vi "Delay.vi"(8 "error in (no error)":errorcluster, 10 "Delay Time (50 ms)":u32=50, 11 "VISA resource name":refnum<visa-resource-name>="TCPIP0::192.168.0.200::50505::SOCKET") -> (0 "error out":errorcluster, 3 "VISA resource name out":refnum<visa-resource-name>="TCPIP0::192.168.0.200::50505::SOCKET")   [LabVIEW 2022 SP3, in "MagnaDC.lvlib"]
uses:
  MagnaDC.lvlib
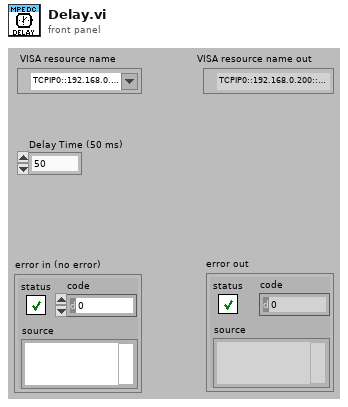
[diagram p1: front panel]
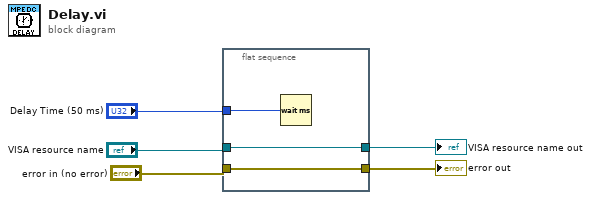
[diagram p0: block diagram]
diagram:
  n1 = flat-sequence {
    tunnel: "Delay Time (50 ms)" -> [w8]
    tunnel: [w7] -> w1
    tunnel: "VISA resource name" -> [w7]
    tunnel: "error in (no error)" -> [w6]
    tunnel: [w6] -> w2
    frame #0 {
      n2 = Wait (ms)(milliseconds to wait=w8) -> ()  [unwired: 1 out]
    }
  }
  "error out" <- w2
  "VISA resource name out" <- w1
